vi "IV-CV-sequence.vi"() -> ()   [LabVIEW 2018]
panel:
  out "Status":string="Press Run to get started."
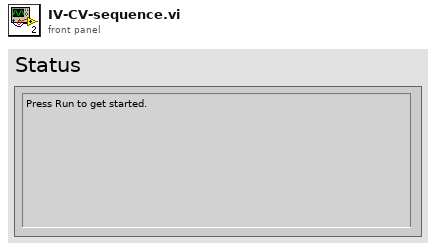
[diagram p1: front panel]
types:
  T1 = enum32{"Invalid", "Standard", "Closed", "Hidden", "Minimized", "Maximized"}
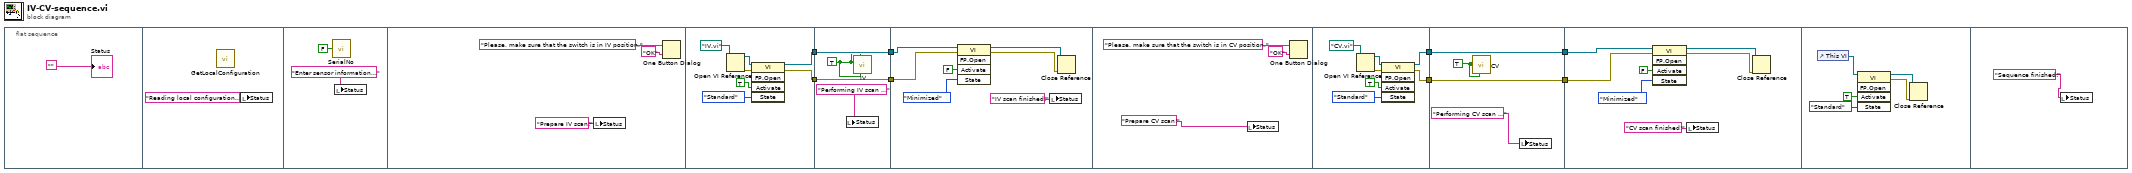
[diagram p0: block diagram]
diagram:
  n1 = flat-sequence {
    tunnel: [w17] -> w7
    tunnel: [w16] -> w5
    tunnel: [w26] -> w8
    tunnel: w7 -> [w26]
    tunnel: [w25] -> w6
    tunnel: w5 -> [w25]
    tunnel: w8 -> [w33]
    tunnel: w6 -> [w32]
    tunnel: [w38] -> w3
    tunnel: [w37] -> w1
    tunnel: [w47] -> w4
    tunnel: w3 -> [w47]
    tunnel: [w46] -> w2
    tunnel: w1 -> [w46]
    tunnel: w4 -> [w50]
    tunnel: w2 -> [w49]
    frame #0 {
      "Status" <- ""
    }
    frame #1 {
      n2 = call "GetLocalConfiguration.vi"() -> ()  [unwired: 3 in, 1 out]
      n3 = local write "Status"("Reading local configuration..." ("Status")) -> ()
    }
    frame #2 {
      n4 = call "SerialNo.vi"("Run uninterrupted?"=FALSE) -> ()  [unwired: 7 in, 2 out]
      n5 = local write "Status"("Enter sensor information..." ("Status")) -> ()
    }
    frame #3 {
      n6 = local write "Status"("Prepare IV scan!" ("Status")) -> ()
      n7 = One Button Dialog(message="Please, make sure that the switch is in IV position.", button name ("OK")="OK") -> ()  [unwired: 1 out]
    }
    frame #4 {
      n8 = Open VI Reference(vi path=path "IV.vi" ("IV path")) -> (vi reference=w21:refnum<vi>, error out=w20:errorcluster)  [unwired: 5 in]
      n9 = invoke class="VI" method="FP.Open"(reference=w21, error in=w20, "Activate"=TRUE ("Activate?"), "State"=T1."Standard") -> (reference out=w16:refnum<vi>, error out=w17:errorcluster)  [unwired: 1 in, 3 out]
    }
    frame #5 {
      w23 = TRUE
      n10 = local write "Status"("Performing IV scan ..." ("Status")) -> ()
      n11 = call "IV.vi"("Run uninterrupted?"=w23, "Wait for continue"=w23, "Sensor info filled?"=w23) -> ()  [unwired: 4 in, 1 out]
    }
    frame #6 {
      n12 = invoke class="VI" method="FP.Open"(reference=w32, error in=w33, "Activate"=FALSE ("Activate?"), "State"=T1."Minimized") -> (reference out=w28:refnum<vi>, error out=w29:errorcluster)  [unwired: 1 in, 3 out]
      n13 = local write "Status"("IV scan finished!" ("Status")) -> ()
      n14 = Close Reference(reference=w28, error in (no error)=w29) -> ()  [unwired: 1 out]
    }
    frame #7 {
      n15 = local write "Status"("Prepare CV scan!" ("Status")) -> ()
      n16 = One Button Dialog(message="Please, make sure that the switch is in CV position.", button name ("OK")="OK") -> ()  [unwired: 1 out]
    }
    frame #8 {
      n17 = Open VI Reference(vi path=path "CV.vi" ("CV path")) -> (vi reference=w42:refnum<vi>, error out=w41:errorcluster)  [unwired: 5 in]
      n18 = invoke class="VI" method="FP.Open"(reference=w42, error in=w41, "Activate"=TRUE ("Activate?"), "State"=T1."Standard") -> (reference out=w37:refnum<vi>, error out=w38:errorcluster)  [unwired: 1 in, 3 out]
    }
    frame #9 {
      w44 = TRUE
      n19 = call "CV.vi"("Run uninterrupted?"=w44, "Wait for continue"=w44, "Sensor info filled?"=w44) -> ()  [unwired: 4 in, 1 out]
      n20 = local write "Status"("Performing CV scan ..." ("Status")) -> ()
    }
    frame #10 {
      n21 = invoke class="VI" method="FP.Open"(reference=w49, error in=w50, "Activate"=FALSE ("Activate?"), "State"=T1."Minimized") -> (reference out=w51:refnum<vi>, error out=w52:errorcluster)  [unwired: 1 in, 3 out]
      n22 = local write "Status"("CV scan finished!" ("Status")) -> ()
      n23 = Close Reference(reference=w51, error in (no error)=w52) -> ()  [unwired: 1 out]
    }
    frame #11 {
      n24 = control-ref of="This VI"() -> (w57:refnum<vi>)
      n25 = invoke class="VI" method="FP.Open"(reference=w57, "Activate"=TRUE ("Activate?"), "State"=T1."Standard") -> (reference out=w58:refnum<vi>, error out=w59:errorcluster)  [unwired: 2 in, 3 out]
      n26 = Close Reference(reference=w58, error in (no error)=w59) -> ()  [unwired: 1 out]
    }
    frame #12 {
      n27 = local write "Status"("Sequence finished!") -> ()
    }
  }
